vi "replaceUniquifier.vi"(8 "error in (no error)":errorcluster, 10 "Query In":string, 11 "Banking Transaction in":refnum<class "Banking Transaction.lvclass">) -> (0 "error out":errorcluster, 2 "Query Out":string, 3 "Banking Transaction out":refnum<class "Banking Transaction.lvclass">)   [LabVIEW 2018, in "Banking Transaction.lvclass"]
uses:
  Banking Transaction.lvclass
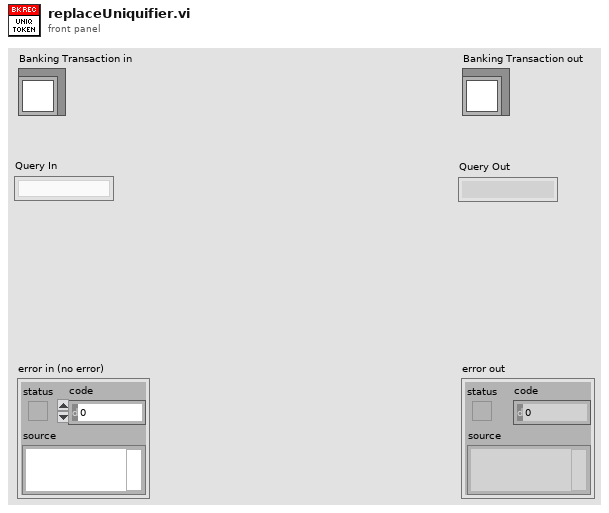
[diagram p1: front panel]
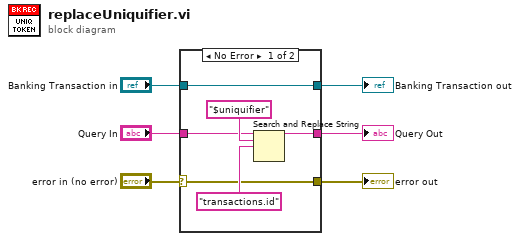
[diagram p0: block diagram]
diagram:
  n1 = case shown="No Error" "error in (no error)" {
    selector: "error in (no error)" -> [w8 w13]
    tunnel: "Query In" -> [w10 w14]
    tunnel: [w9 w14] -> w5
    tunnel: [w8 w13] -> w3
    tunnel: "Banking Transaction in" -> [w7 w15]
    tunnel: [w7 w15] -> w1
    frame No Error {
      n2 = Search and Replace String(input string=w10, search string="$uniquifier", replace string="transactions.id") -> (result string=w9:string)  [unwired: 5 in, 3 out]
    }
    frame Error {
    }
  }
  "error out" <- w3
  "Banking Transaction out" <- w1
  "Query Out" <- w5
